vi "Set_NextObj_properties.vi"(0 "Target RA":dbl format="%<%H:%M:%S%1u>t", 7 "Target DEC":dbl format="%<%H:%M:%S>t", 11 "Target Epoch":dbl format="%.3g", 13 "Sideral Time":dbl format="%<%H:%M:%S>t") -> (4 "NO RA":string, 6 "NO DEC":string, 8 "NO Epoch":dbl, 10 "NO HA":dbl format="%<%H:%M:%S>t", 15 "NO AM":dbl)   [LabVIEW 2011]
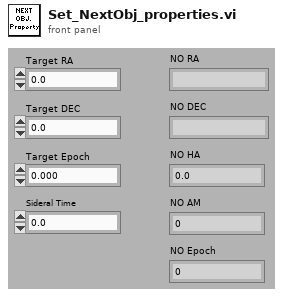
[diagram p1: front panel]
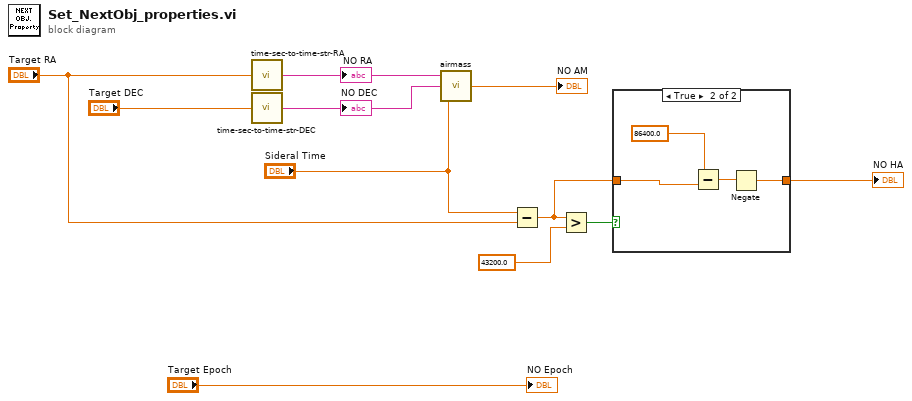
[diagram p0: block diagram]
diagram:
  n1 = call "time-sec-to-time-str-RA.vi"("Numeric"="Target RA") -> ("formatted-str"=w10:string)
  "NO RA" <- w10
  n2 = call "time-sec-to-time-str-DEC.vi"("Numeric"="Target DEC") -> ("formatted-str"=w9:string)
  "NO DEC" <- w9
  n3 = call "airmass.vi"("temps sidéral"="Sideral Time", "DEC"=w9, "RA"=w10) -> ("airmass"=→"NO AM":dbl)
  n4 = Subtract(x="Sideral Time", y="Target RA") -> (x-y=w2:dbl)
  n5 = Greater?(x=w2, y=43200.0) -> (0:w3:bool)
  n6 = case shown="True" w3 {
    tunnel: w2 -> [w12 w16]
    tunnel: [w12 w14] -> w1
    frame False {
    }
    frame True {
      n7 = Subtract(x=86400.0, y=w16) -> (x-y=w15:dbl)
      n8 = Negate(x=w15) -> (-x=w14:dbl)
    }
  }
  "NO HA" <- w1
  "NO Epoch" <- "Target Epoch"
